vi "Pad out Mapping.vi"(7 "PDO Mappables":string[](array[string]), 8 "error in":errorcluster, 9 "Bit Offset":i32, 10 "Row":i32, 11 "PDO Grid in":refnum<class "PDO Grid.lvclass">) -> (0 "error out":errorcluster, 3 "PDO Grid out":refnum<class "PDO Grid.lvclass">)   [LabVIEW 2019, in "PDO Grid.lvlib" / "PDO Grid.lvclass"]
uses:
  PDO Grid.lvclass
  D:/git/Sourcegrid-LabVIEW/source/Grid/SourceGrid.lvclass
  Sourcegrid-LabVIEW/source/Cells/Cell/Cell.lvclass
  Sourcegrid-LabVIEW/source/Editors/Combo Box/Combo Box.lvclass
  D:/git/Sourcegrid-LabVIEW/source/Editors/Editor Base/Editor Control Base.lvclass
  Sourcegrid-LabVIEW/source/Views/Cell View Alternating Back Color/Cell View Alternating Back Color.lvclass
  D:/git/Sourcegrid-LabVIEW/source/Views/Cell View/Cell View.lvclass
  Sourcegrid-LabVIEW/source/System.Drawing.Color.ctl
  Sourcegrid-LabVIEW/source/SourceGrid.lvlib
  Sourcegrid-LabVIEW/source/Grid/SourceGrid.lvclass
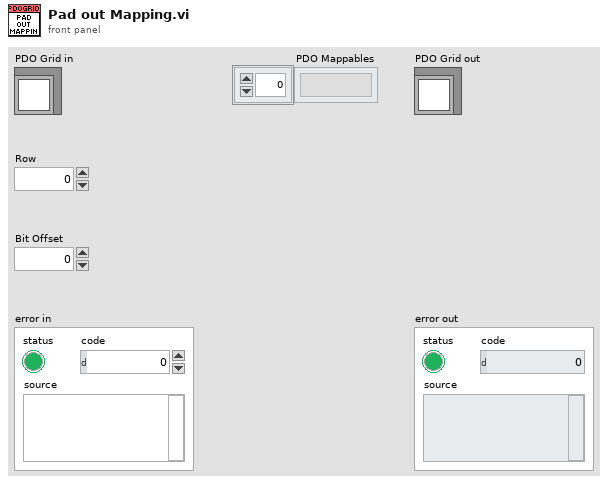
[diagram p1: front panel]
types:
  T1 = typedef "SourceGrid.lvlib/System.Drawing.Color.ctl" = enum16{"AliceBlue", "AntiqueWhite", "Aqua", "Aquamarine", "Azure", "Beige", "Bisque", "Black", "BlanchedAlmond", "Blue", "BlueViolet", "Brown", "BurlyWood", "CadetBlue", "Chartreuse", "Chocolate", "Coral", "CornflowerBlue", "Cornsilk", "Crimson", "Cyan", "DarkBlue", "DarkCyan", "DarkGoldenrod", "DarkGray", "DarkGreen", "DarkKhaki", "DarkMagenta", "DarkOliveGreen", "DarkOrange", "DarkOrchid", "DarkRed", "DarkSalmon", "DarkSeaGreen", "DarkSlateBlue", "DarkSlateGray", "DarkTurquoise", "DarkViolet", "DeepPink", "DeepSkyBlue", "DimGray", "DodgerBlue", "Firebrick", "FloralWhite", "ForestGreen", "Fuchsia", "Gainsboro", "GhostWhite", "Gold", "Goldenrod", "Gray", "Green", "GreenYellow", "Honeydew", "HotPink", "IndianRed", "Indigo", "Ivory", "Khaki", "Lavender", "LavenderBlush", "LawnGreen", "LemonChiffon", "LightBlue", "LightCoral", "LightCyan", "LightGoldenrodYellow", "LightGray", "LightGreen", "LightPink", "LightSalmon", "LightSeaGreen", "LightSkyBlue", "LightSlateGray", "LightSteelBlue", "LightYellow", "Lime", "LimeGreen", "Linen", "Magenta", "Maroon", "MediumAquamarine", "MediumBlue", "MediumOrchid", "MediumPurple", "MediumSeaGreen", "MediumSlateBlue", "MediumSpringGreen", "MediumTurquoise", "MediumVioletRed", "MidnightBlue", "MintCream", "MistyRose", "Moccasin", "NavajoWhite", "Navy", "OldLace", "Olive", "OliveDrab", "Orange", "OrangeRed", "Orchid", "PaleGoldenrod", "PaleGreen", "PaleTurquoise", "PaleVioletRed", "PapayaWhip", "PeachPuff", "Peru", "Pink", "Plum", "PowderBlue", "Purple", "Red", "RosyBrown", "RoyalBlue", "SaddleBrown", "Salmon", "SandyBrown", "SeaGreen", "SeaShell", "Sienna", "Silver", "SkyBlue", "SlateBlue", "SlateGray", "Snow", "SpringGreen", "SteelBlue", "Tan", "Teal", "Thistle", "Tomato", "Transparent", "Turquoise", "Violet", "Wheat", "White", "WhiteSmoke", "Yellow"}
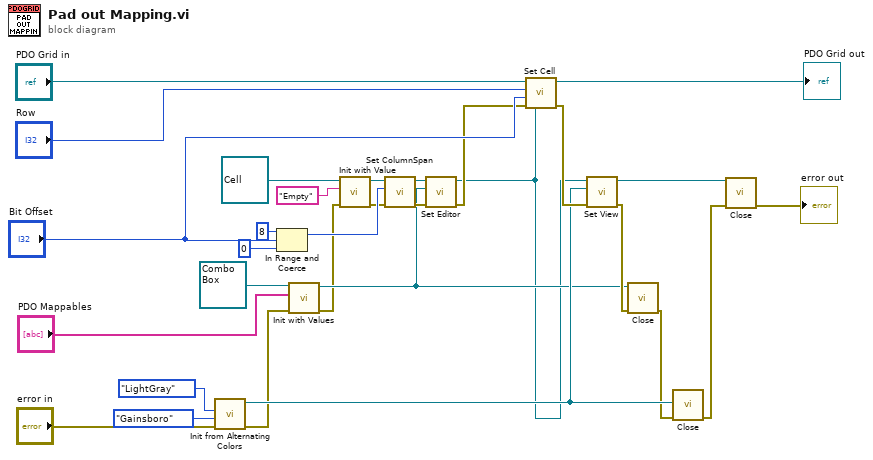
[diagram p0: block diagram]
diagram:
  n1 = call "Init from Alternating Colors.vi"("error in"="error in", "Color Not Equal"=System.Drawing.Color."Gainsboro", "Color Equal"=System.Drawing.Color."LightGray" ("Color")) -> ("error out"=w2:errorcluster, "Cell View Alternating Back Color out"=w11:refnum<class "Cell View Alternating Back Color.lvclass">)  [unwired: 7 in]
  n2 = In Range and Coerce(upper limit=8 ("y"), x="Bit Offset", lower limit=0) -> (coerced(x)=w25:i32)  [unwired: 1 out]
  n3 = call-dynamic "Init with Values.vi"("error in"=w2, "Values"="PDO Mappables", "Combo Box in"=refnum<class "Combo Box.lvclass"> refnum ("SourceGrid.lvlib:Combo Box.lvclass")) -> ("error out"=w1:errorcluster, "Combo Box out"=w4:refnum<class "Combo Box.lvclass">)  [unwired: 7 in]
  n4 = call-dynamic "Init with Value.vi"("error in"=w1, "Value"="Empty", "Cell in"=refnum<class "Cell.lvclass"> refnum ("SourceGrid.lvlib:Cell.lvclass")) -> ("error out"=w23:errorcluster, "Cell out"=w24:refnum<class "Cell.lvclass">)  [unwired: 7 in]
  n5 = call "Set ColumnSpan.vi"("error in"=w23, "ColumnSpan"=w25, "Cell in"=w24) -> ("error out"=w10:errorcluster, "Cell out"=w28:refnum<class "Cell.lvclass">)  [unwired: 7 in]
  n6 = call-dynamic "Set Editor.vi"("error in"=w10, "Editor Control Base"=w4, "Cell in"=w28) -> ("error out"=w9:errorcluster, "Cell out"=w3:refnum<class "Cell.lvclass">)  [unwired: 7 in]
  n7 = call "Set Cell.vi"("Cell"=w3, "error in"=w9, "Column"="Bit Offset", "Row"="Row", "Sourcegrid in"="PDO Grid in") -> ("error out"=w12:errorcluster, "Sourcegrid out"=→"PDO Grid out":refnum<class "PDO Grid.lvclass">)  [unwired: 5 in]
  n8 = call-dynamic "Set View.vi"("error in"=w12, "CellView"=w11, "Cell in"=w3) -> ("error out"=w6:errorcluster, "Cell out"=w13:refnum<class "Cell.lvclass">)  [unwired: 7 in]
  n9 = call-dynamic "Close.vi"("error in"=w6, "Combo Box in"=w4) -> ("error out"=w5:errorcluster)  [unwired: 8 in, 1 out]
  n10 = call-dynamic "Close.vi"("error in"=w5, "Cell View Alternating Back Color in"=w11) -> ("error out"=w27:errorcluster)  [unwired: 8 in, 1 out]
  n11 = call-dynamic "Close.vi"("error in"=w27, "Cell in"=w13) -> ("error out"=→"error out":errorcluster)  [unwired: 8 in, 1 out]
